vi "CLC_JIO_INIT.vi"(7 "Func.":enum16{"ALL", "BFIC", "UDIC", "OFF"}(ring), 8 "error in":errorcluster) -> (0 "error out":errorcluster, 3 "standard output":string)   [LabVIEW 2023, in "CLC_JIO_FTDI.lvlib"]
uses:
  CLC_JIO_FTDI.lvlib
panel:
  out "standard error":string
  out "floder?":bool
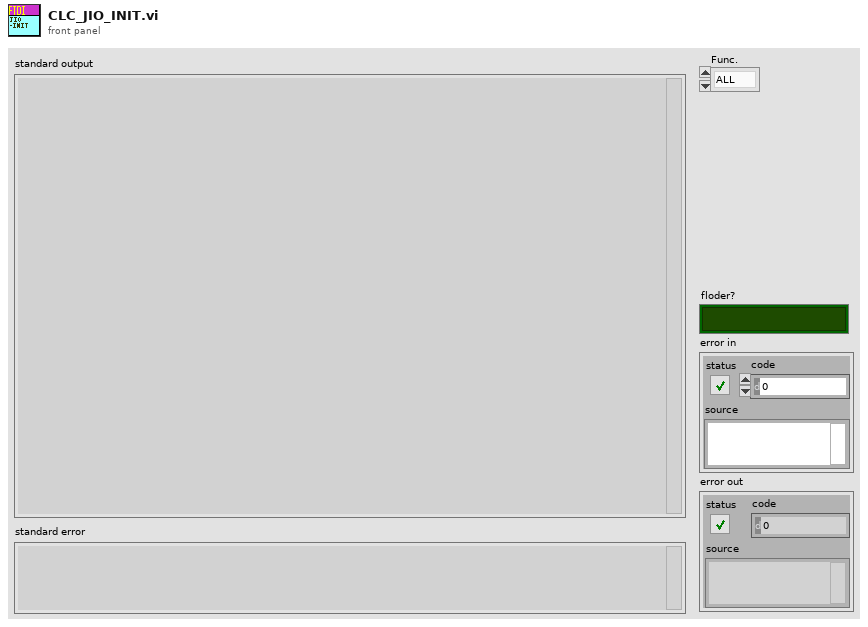
[diagram p1: front panel]
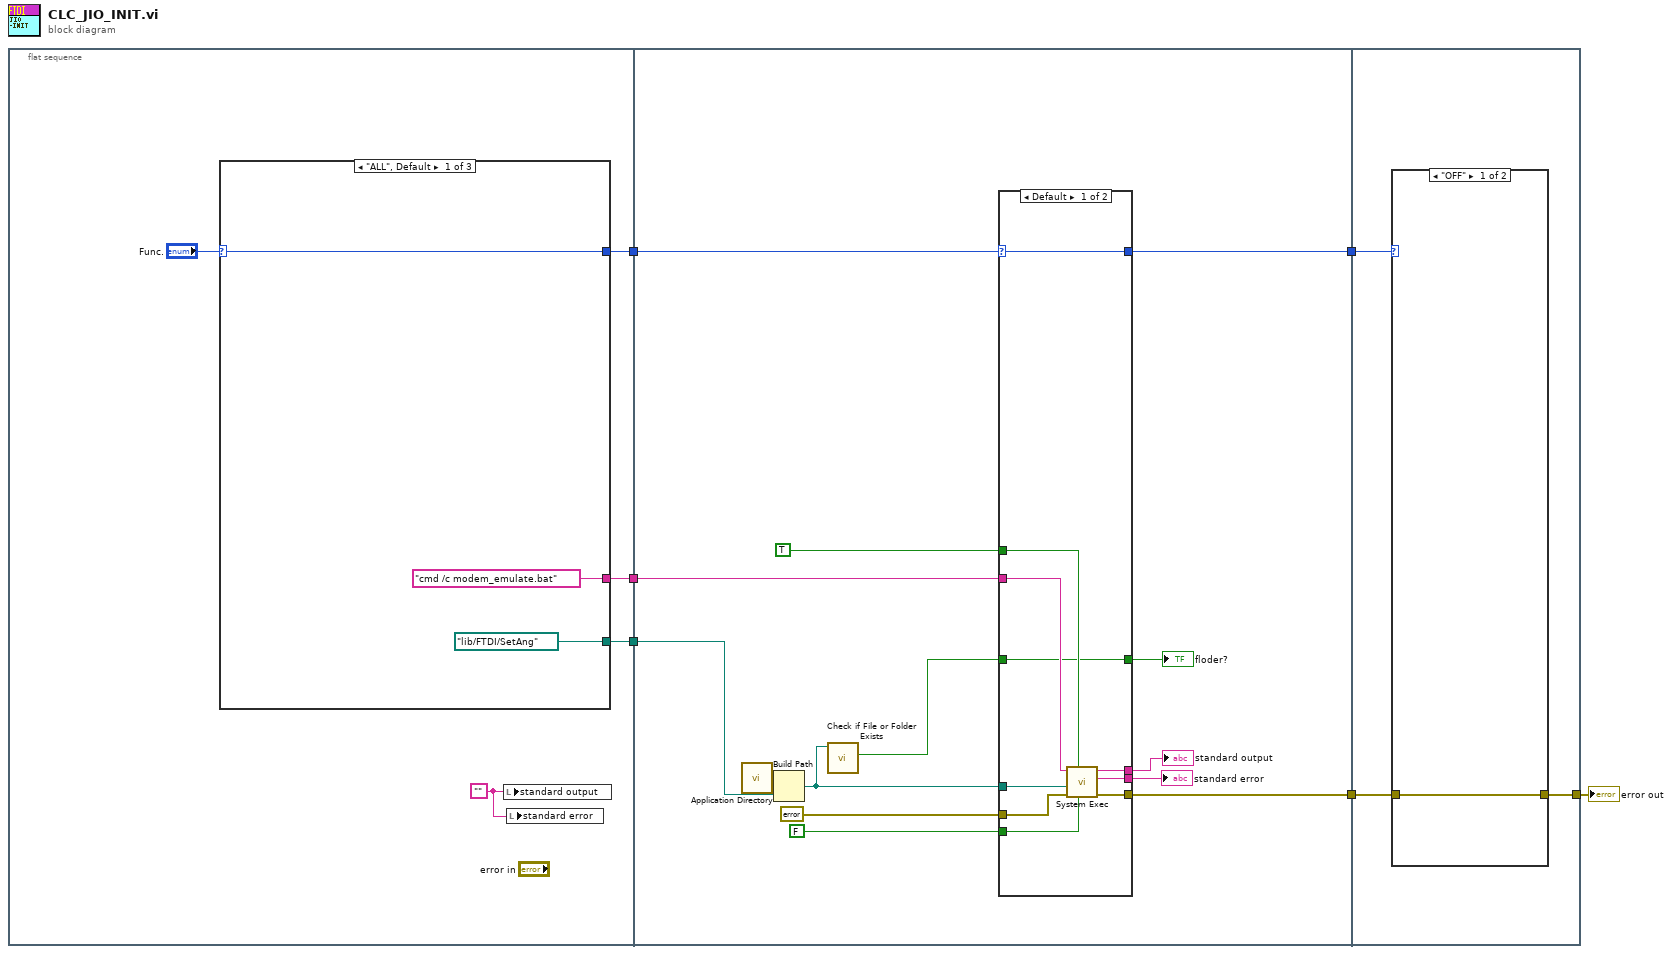
[diagram p0: block diagram]
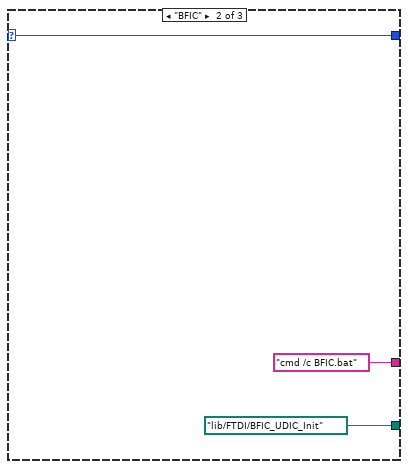
[diagram p2: hidden frame]
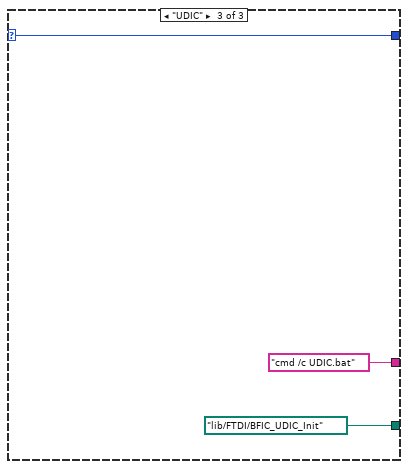
[diagram p3: hidden frame]
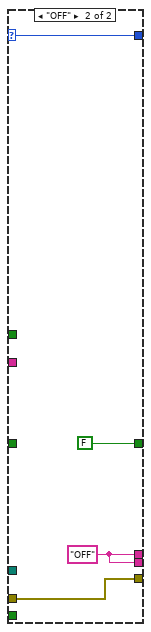
[diagram p4: hidden frame]
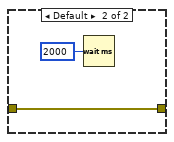
[diagram p5: hidden frame]
diagram:
  n1 = flat-sequence {
    tunnel: [w10] -> w4
    tunnel: [w9] -> w3
    tunnel: [w7] -> w1
    tunnel: [w28] -> w5
    tunnel: w4 -> [w26]
    tunnel: w3 -> [w25]
    tunnel: [w21] -> w2
    tunnel: w1 -> [w24]
    tunnel: [w50] -> w6
    tunnel: w5 -> [w51]
    tunnel: w2 -> [w49]
    frame #0 {
      w11 = ""
      n2 = case shown="\"ALL\", Default" "Func." {
        selector: "Func." -> [w12 w15 w18]
        tunnel: ["cmd /c modem_emulate.bat" ("command line") "cmd /c BFIC.bat" ("command line") "cmd /c UDIC.bat" ("command line")] -> w10
        tunnel: [path "lib/FTDI/SetAng" ("name or relative path") path "lib/FTDI/BFIC_UDIC_Init" ("name or relative path") path "lib/FTDI/BFIC_UDIC_Init" ("name or relative path")] -> w9
        tunnel: [w12 w15 w18] -> w7
        frame "ALL", Default {
        }
        frame "BFIC" {
        }
        frame "UDIC" {
        }
      }
      n3 = local write "standard output"(w11) -> ()
      n4 = local write "standard error"(w11) -> ()
    }
    frame #1 {
      n5 = call <vilib>:"Application Directory.vi"() -> ("Application Directory"=w31:path)
      n6 = Build Path(base path=w31, name or relative path=w25) -> (appended path=w34:path)
      n7 = call <vilib>:"Check if File or Folder Exists.vi"("path"=w34) -> ("file or folder exists?"=w23:bool)  [unwired: 8 in, 2 out]
      n8 = case shown="Default" w24 {
        selector: w24 -> [w35 w45]
        tunnel: w34 -> [w44 _]
        tunnel: [w43 w46] -> w33
        tunnel: [w42 w46] -> w32
        tunnel: FALSE ("run minimized? (F)") -> [w41 _]
        tunnel: TRUE ("wait until completion? (T)") -> [w40 _]
        tunnel: [w39 w48] -> w28
        tunnel: errorcluster {"status"=FALSE, "code"=0, "source"=""} ("error in (no error)") -> [w38 w48]
        tunnel: w26 -> [w37 _]
        tunnel: w23 -> [w36 _]
        tunnel: [w36 FALSE ("file or folder exists?")] -> w22
        tunnel: [w35 w45] -> w21
        frame Default {
          n9 = call <vilib>:"System Exec.vi"("run minimized? (F)"=w41, "wait until completion? (T)"=w40, "error in (no error)"=w38, "working directory"=w44, "command line"=w37) -> ("error out"=w39:errorcluster, "standard error"=w43:string, "standard output"=w42:string)  [unwired: 3 in, 1 out]
        }
        frame "OFF" {
          w46 = "OFF"
        }
      }
      "floder?" <- w22
      "standard output" <- w32
      "standard error" <- w33
    }
    frame #2 {
      n10 = case shown="\"OFF\"" w49 {
        tunnel: w51 -> [w52 w53]
        tunnel: [w52 w53] -> w50
        frame "OFF" {
        }
        frame Default {
          n11 = Wait (ms)(milliseconds to wait=u32 2000) -> ()  [unwired: 1 out]
        }
      }
    }
  }
  "error out" <- w6
